vi "Set_WindDir_Calibration.vi"(1 "Wind dir offset":i32, 2 "Path":path) -> (0 "Calibration value set?":bool)   [LabVIEW 2013]
uses:
  <vilib>/Utility/config.llb/Write Key (I32).vi
  VantagePro.dll
  <vilib>/Utility/config.llb/NI_LVConfig.lvlib
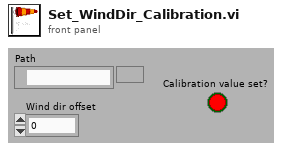
[diagram p1: front panel]
types:
  T1 = typedef "NI_LVConfig.lvlib/Config Data RefNum.ctl" = refnum<k1>
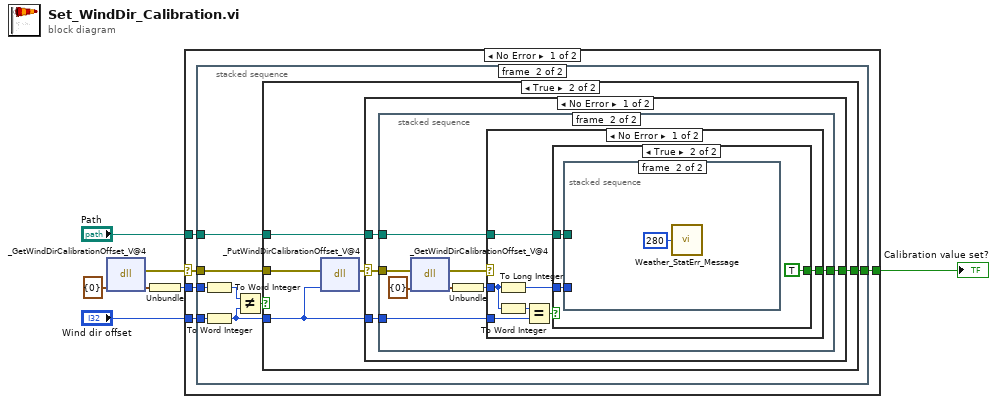
[diagram p0: block diagram]
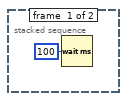
[diagram p2: hidden frame]
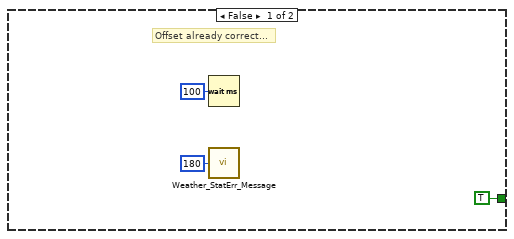
[diagram p3: hidden frame]
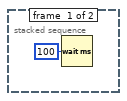
[diagram p4: hidden frame]
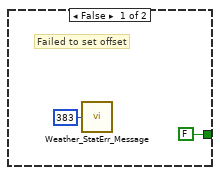
[diagram p5: hidden frame]
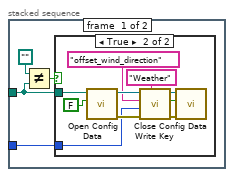
[diagram p6: hidden frame]
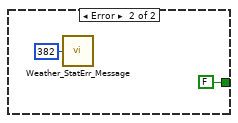
[diagram p8: hidden frame]
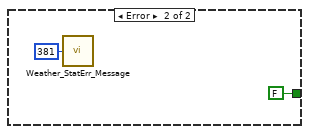
[diagram p9: hidden frame]
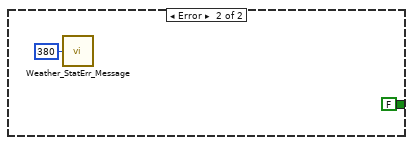
[diagram p10: hidden frame]
diagram:
  n1 = dll-call lib="C:/Users/Bob van Eijk/Desktop/LabView Projects 13/HiSPARC Weather Station/Develop/VantagePro.dll" fn="_GetWindDirCalibrationOffset_V@4" label="Get wind dir offset"("winddirectionoff"=cluster{i16} {0}) -> (error out=w2:errorcluster, "winddirectionoff"=w4:cluster{i16})  [unwired: 4 in, 1 out]
  n2 = Unbundle(w4) -> (w1:i16)
  n3 = case shown="No Error" w2 {
    selector: w2 -> [w10 _]
    tunnel: "Path" -> [w12 _]
    tunnel: [w8 FALSE] -> w5
    tunnel: w1 -> [w9 _]
    tunnel: "Wind dir offset" -> [w11 _]
    frame No Error {
      n4 = stacked-sequence {
        tunnel: w12 -> [_ w21]
        tunnel: w11 -> [_ w20]
        tunnel: w10 -> [_ w18]
        tunnel: w9 -> [_ w16]
        tunnel: [_ w15] -> w8
        frame #0 {
          n5 = Wait (ms)(milliseconds to wait=u32 100) -> ()  [unwired: 1 out]
        }
        frame #1 {
          n6 = To Word Integer(number=w16) -> (16bit integer=w14:i16)
          n7 = To Word Integer(number=w20) -> (16bit integer=w17:i16)
          n8 = Not Equal?(x=w14, y=w17) -> (x != y?=w19:bool)
          n9 = case shown="True" w19 {
            tunnel: w21 -> [_ w28]
            tunnel: [TRUE w29] -> w15
            tunnel: w18 -> [_ w27]
            tunnel: w17 -> [_ w25]
            frame False {
              # "Offset already correct..."
              n10 = Wait (ms)(milliseconds to wait=u32 100) -> ()  [unwired: 1 out]
              n11 = call "Weather_StatErr_Message.vi"("Message number"=180) -> ()  [unwired: 1 out]
            }
            frame True {
              n12 = dll-call lib="C:/Users/Bob van Eijk/Desktop/LabView Projects 13/HiSPARC Weather Station/Develop/VantagePro.dll" fn="_PutWindDirCalibrationOffset_V@4" label="Set wind dir offset"(error in=w27, "winddirectionoff"=w25) -> (error out=w26:errorcluster)  [unwired: 4 in, 1 out]
              n13 = case shown="No Error" w26 {
                selector: w26 -> [w30 _]
                tunnel: [w33 FALSE] -> w29
                tunnel: w28 -> [w32 _]
                tunnel: w25 -> [w31 _]
                frame No Error {
                  n14 = stacked-sequence {
                    tunnel: w32 -> [_ w42]
                    tunnel: [_ w41] -> w33
                    tunnel: w31 -> [_ w40]
                    tunnel: w30 -> [_ w39]
                    frame #0 {
                      n15 = Wait (ms)(milliseconds to wait=u32 100) -> ()  [unwired: 1 out]
                    }
                    frame #1 {
                      n16 = dll-call lib="C:/Users/Bob van Eijk/Desktop/LabView Projects 13/HiSPARC Weather Station/Develop/VantagePro.dll" fn="_GetWindDirCalibrationOffset_V@4" label="Get wind dir offset"(error in=w39, "winddirectionoff"=cluster{i16} {0}) -> (error out=w35:errorcluster, "winddirectionoff"=w38:cluster{i16})  [unwired: 3 in, 1 out]
                      n17 = Unbundle(w38) -> (w36:i16)
                      n18 = case shown="No Error" w35 {
                        tunnel: w42 -> [w49 _]
                        tunnel: [w48 FALSE] -> w41
                        tunnel: w36 -> [w47 _]
                        tunnel: w40 -> [w46 _]
                        frame No Error {
                          n19 = To Long Integer(number=w47) -> (32bit integer=w44:i32)
                          n20 = To Word Integer(number=w47) -> (16bit integer=w45:i16)
                          n21 = Equal?(x=w45, y=w46) -> (x = y?=w43:bool)
                          n22 = case shown="True" w43 {
                            tunnel: w49 -> [_ w53]
                            tunnel: w44 -> [_ w54]
                            tunnel: [FALSE TRUE] -> w48
                            frame False {
                              # "Failed to set offset"
                              n23 = call "Weather_StatErr_Message.vi"("Message number"=383) -> ()  [unwired: 1 out]
                            }
                            frame True {
                              n24 = stacked-sequence {
                                tunnel: w54 -> [w58 _]
                                tunnel: w53 -> [w56 _]
                                frame #0 {
                                n25 = Not Equal?(x=path "", y=w56) -> (x != y?=w57:bool)
                                n26 = case shown="True" w57 {
                                tunnel: w58 -> [_ w59]
                                tunnel: w56 -> [_ w60]
                                frame False {
                                }
                                frame True {
                                n27 = call <vilib>:"Open Config Data.vi"("create file if necessary (T)"=FALSE, "configuration file path"=w60) -> ("error out"=w68:errorcluster, "refnum"=w67:T1)  [unwired: 7 in, 1 out]
                                n28 = call-poly <vilib>:"Write Key.vi"("section"="Weather" ("key"), "error in (no error)"=w68, "value"=w59, "key"="offset_wind_direction", "refnum"=w67) -> ("error out"=w66:errorcluster, "found?"=w65:bool, "refnum out"=w64:T1)  [unwired: 4 in]
                                n29 = call <vilib>:"Close Config Data.vi"("error in (no error)"=w66, "write file if changed (T)"=w65, "refnum"=w64) -> ()  [unwired: 7 in, 2 out]
                                }
                                }
                                }
                                frame #1 {
                                n30 = call "Weather_StatErr_Message.vi"("Message number"=280) -> ()  [unwired: 1 out]
                                }
                              }
                            }
                          }
                        }
                        frame Error {
                          n31 = call "Weather_StatErr_Message.vi"("Message number"=382) -> ()  [unwired: 1 out]
                        }
                      }
                    }
                  }
                }
                frame Error {
                  n32 = call "Weather_StatErr_Message.vi"("Message number"=381) -> ()  [unwired: 1 out]
                }
              }
            }
          }
        }
      }
    }
    frame Error {
      n33 = call "Weather_StatErr_Message.vi"("Message number"=380) -> ()  [unwired: 1 out]
    }
  }
  "Calibration value set?" <- w5
